vi "Stops.vi"() -> ()   [LabVIEW 2019]
panel:
  in  "StopPolar":bool
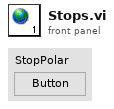
[diagram p1: front panel]
diagram:
